vi "ReadAirmarData.vi"(8 "Error in":errorcluster, 9 "Airmar Wind Queue Cluster":T2, 10 "AirmarGPS-Compass Queue Cluster":T3, 11 "VISA UART port":refnum<visa-resource-name>) -> (0 "Error out":errorcluster, 3 "read buffer":string)   [LabVIEW 2013]
doc: "This VI reads Airmar data from the serial port, extracts the data of relevance, and writes the data to the proper queues for filtering and notification.\n\nEric Schneider, March 2014"
uses:
  Data/TypeDefs/GPS-Compass Queue Cluster.ctl
  Data/TypeDefs/UTM Location.ctl
  Data/TypeDefs/WindData Queue Cluster.ctl
  Data/TypeDefs/Notifiers.ctl
  Data/TypeDefs/Sail Set Suggestions.ctl
  Data/TypeDefs/Rudder Set Suggestions.ctl
  Data/TypeDefs/OverrideInformation.ctl
  Data/TypeDefs/OverrideMode.ctl
  Data/TypeDefs/MotorSetup.ctl
  Data/TypeDefs/DynamixelSetupInfo.ctl
  Data/TypeDefs/AirmarStatus.ctl
  Data/TypeDefs/HardwareOnline.ctl
panel:
  in  "Notifier References":T1
  out "Longitude [deg]":string
  out "Latitude [deg]":string
  in  "time zone":i32
  out "Time":string
  out "Mode":string
  out "Date [ddmmyy]":string
  out "Course over ground [degrees]":string
  out "Status":string
  out "Speed over ground [knots]":string
  out "E/W":string
  out "Longitude":string
  out "N/S":string
  out "Latitude":string
  out "UTC Time":string
  out "NMEA sentences":string
  # "[hhmmss.sss]"
  # "A = vAlid data\nV = inValid data"
  # "[ddmm.mmmm]"
  # "[dddmm.mmmm]"
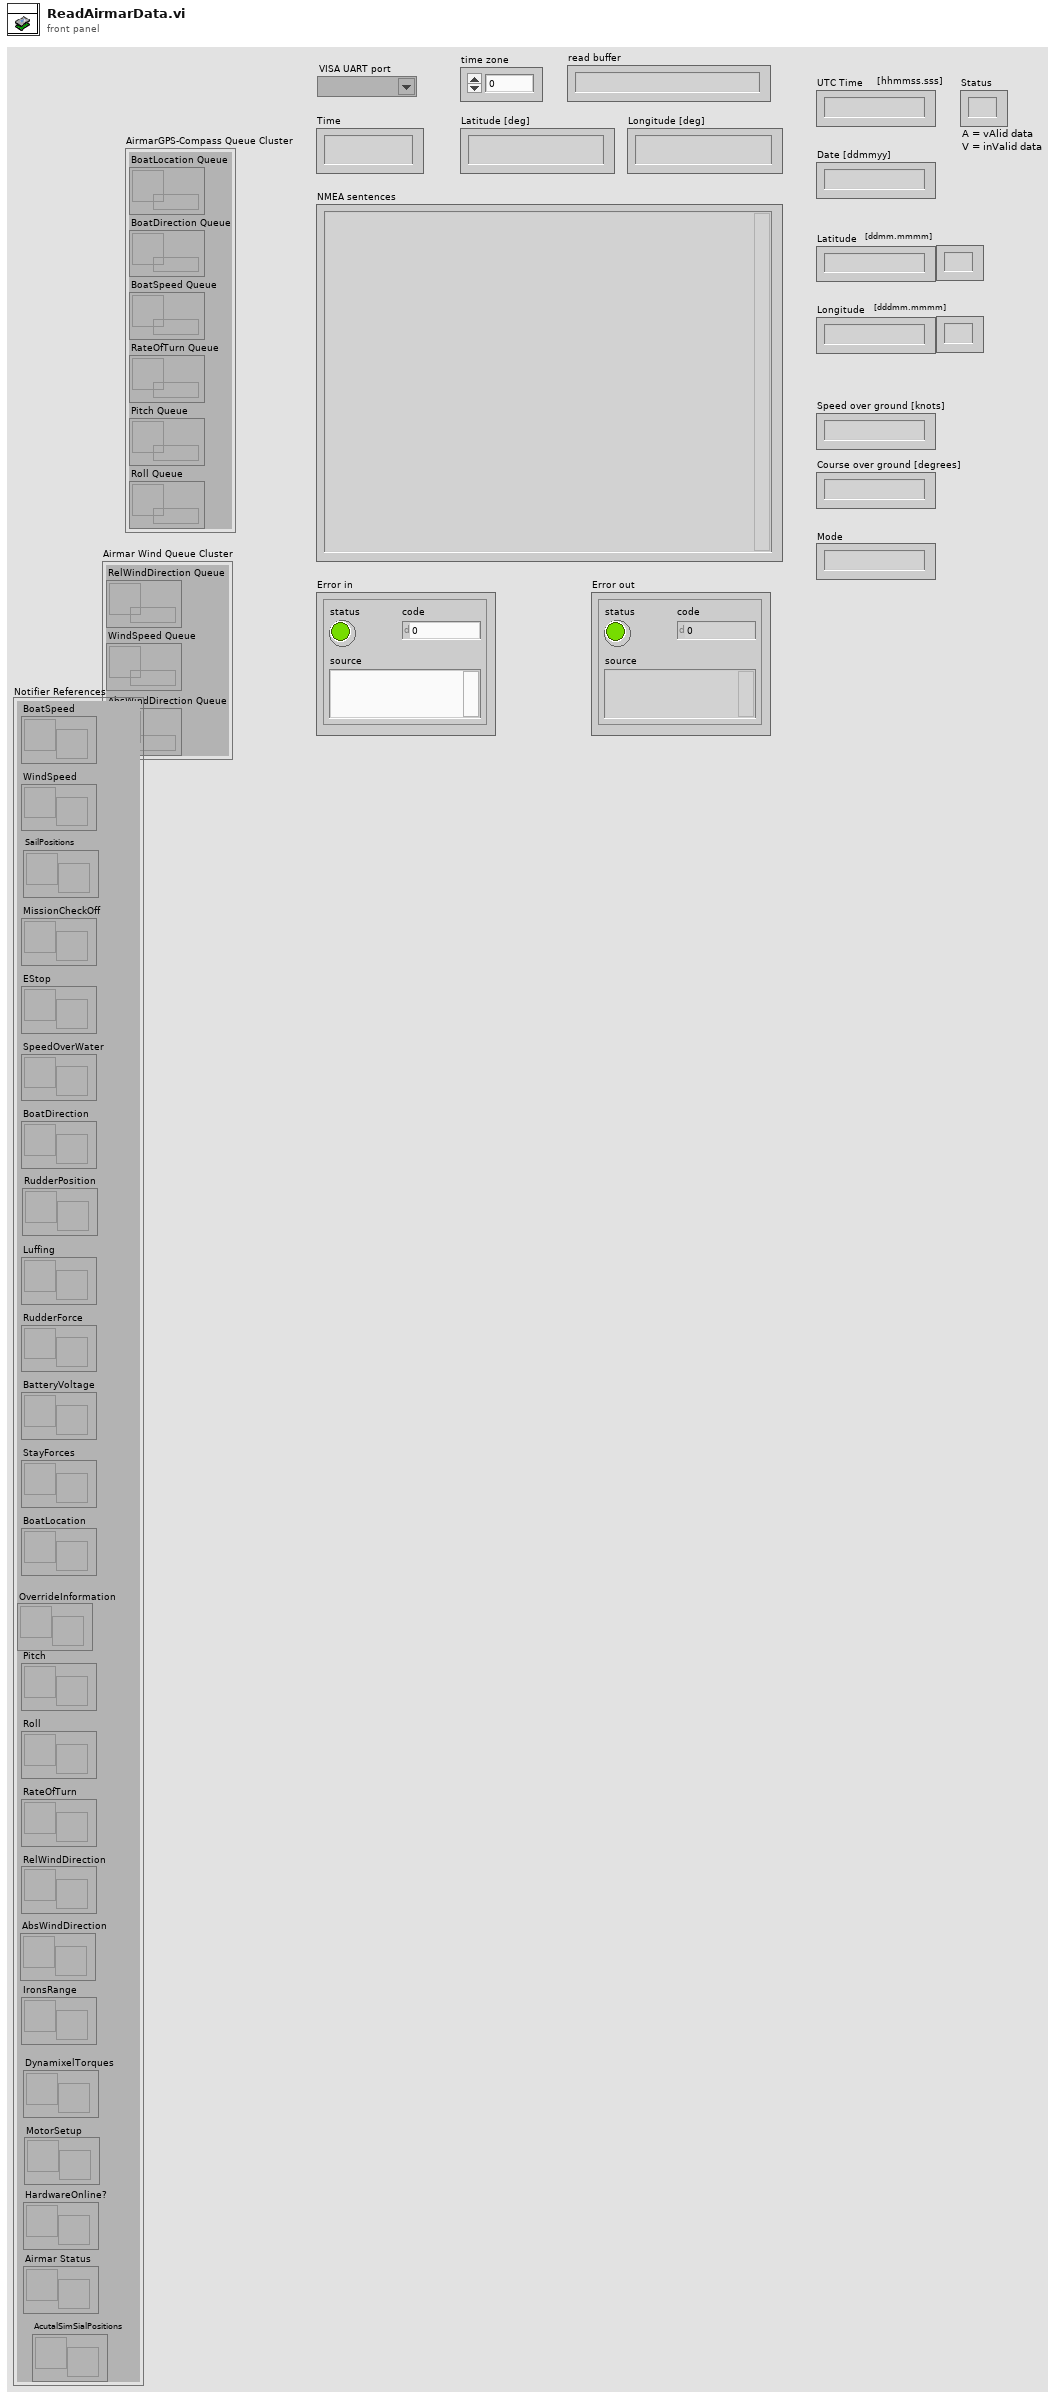
[diagram p1: front panel]
types:
  T1 = typedef "Notifiers.ctl" = cluster{"BoatSpeed":refnum<notifier>, "WindSpeed":refnum<notifier>, "MissionCheckOff":refnum<notifier>, "EStop":refnum<notifier>, "SpeedOverWater":refnum<notifier>, "BoatDirection":refnum<notifier>, "Luffing":refnum<notifier>, "RudderForce":refnum<notifier>, "BatteryVoltage":refnum<notifier>, "StayForces":refnum<notifier>, "BoatLocation":refnum<notifier>, "Pitch":refnum<notifier>, "Roll":refnum<notifier>, "RateOfTurn":refnum<notifier>, "RelWindDirection":refnum<notifier>, "SailPositions":refnum<notifier>, "RudderPosition":refnum<notifier>, "IronsRange":refnum<notifier>, "AbsWindDirection":refnum<notifier>, "OverrideInformation":refnum<notifier>, "DynamixelTorques":refnum<notifier>, "MotorSetup":refnum<notifier>, "Airmar Status":refnum<notifier>, "HardwareOnline?":refnum<notifier>, "AcutalSimSialPositions":refnum<notifier>}
  T2 = typedef "WindData Queue Cluster.ctl" = cluster{"RelWindDirection Queue":refnum<queue>, "WindSpeed Queue":refnum<queue>, "AbsWindDirection Queue":refnum<queue>}
  T3 = typedef "GPS-Compass Queue Cluster.ctl" = cluster{"BoatLocation Queue":refnum<queue>, "BoatDirection Queue":refnum<queue>, "BoatSpeed Queue":refnum<queue>, "RateOfTurn Queue":refnum<queue>, "Pitch Queue":refnum<queue>, "Roll Queue":refnum<queue>}
  T4 = typedef "AirmarStatus.ctl" = cluster{"Sensor Connected":bool, "Sensor Initialized":bool, "Sensor OK":bool, "Latest Error String":bool, "GPS Lock":bool}
  T5 = typedef "UTM Location.ctl" = cluster{"UTM Zone":dbl, "Hemisphere":enum16{"North", "South"}, "East":dbl, "North":dbl}
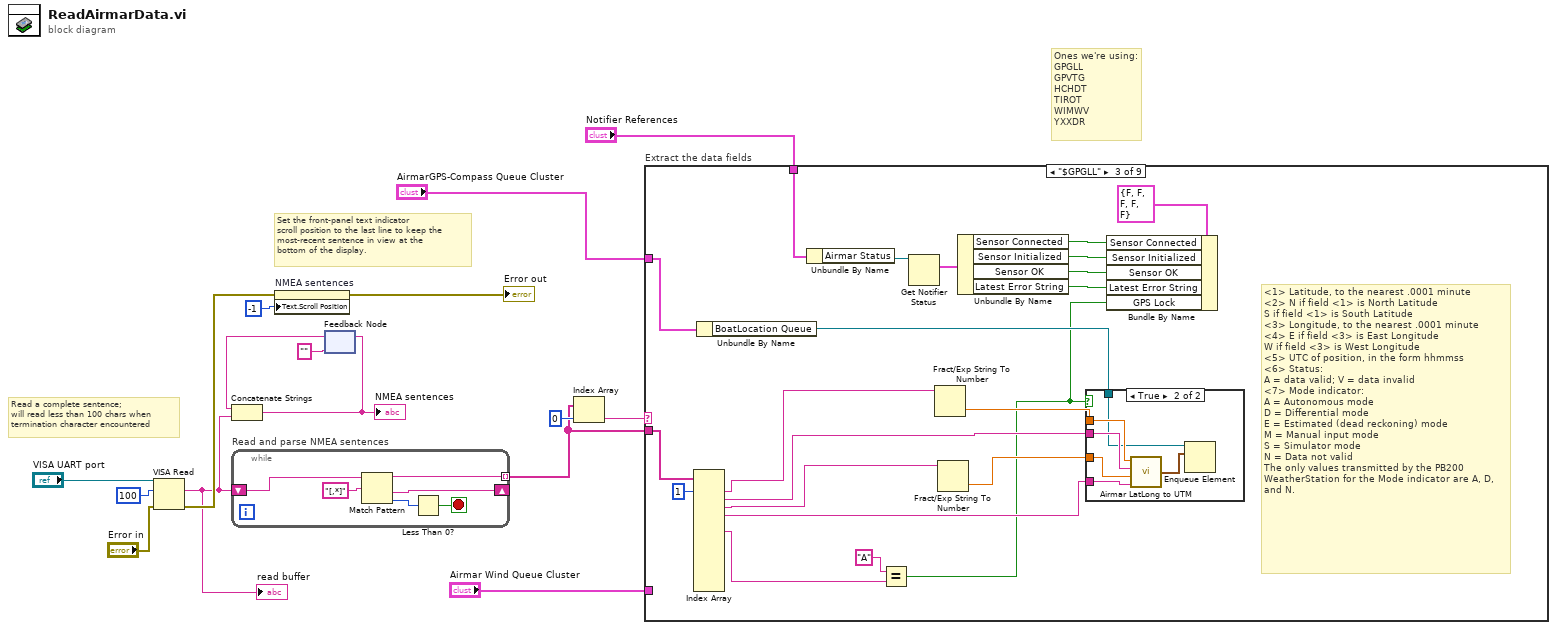
[diagram p0: block diagram]
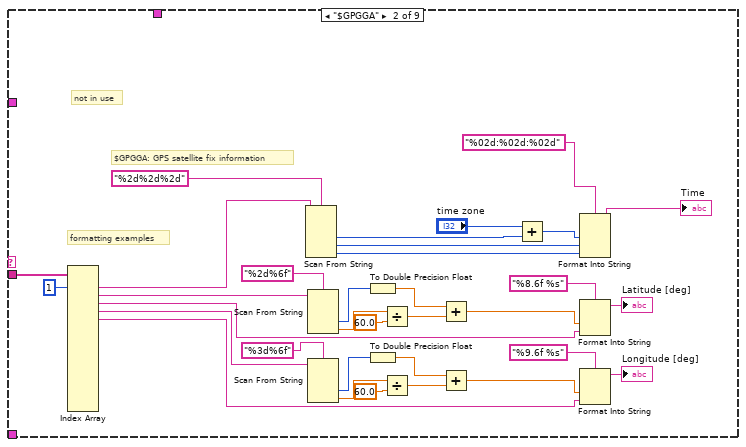
[diagram p3: hidden frame]
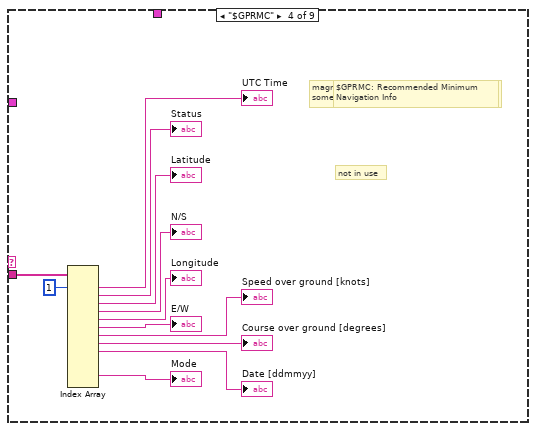
[diagram p5: hidden frame]
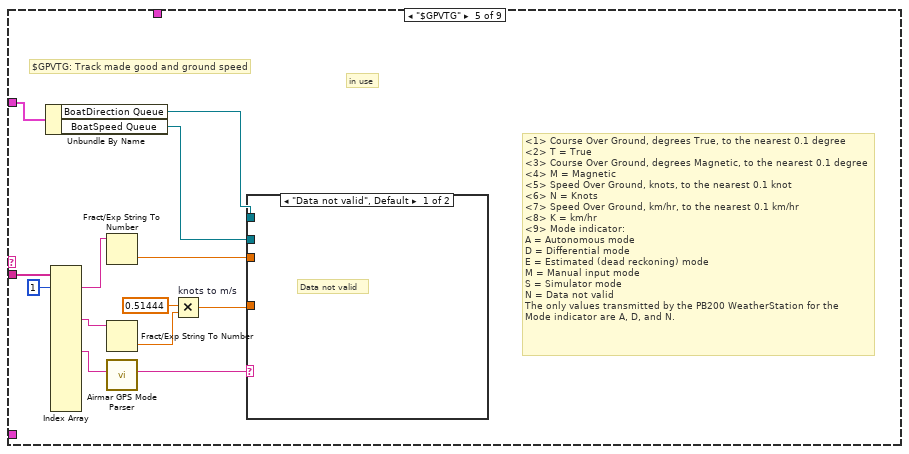
[diagram p6: hidden frame]
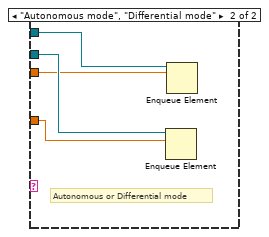
[diagram p7: hidden frame]
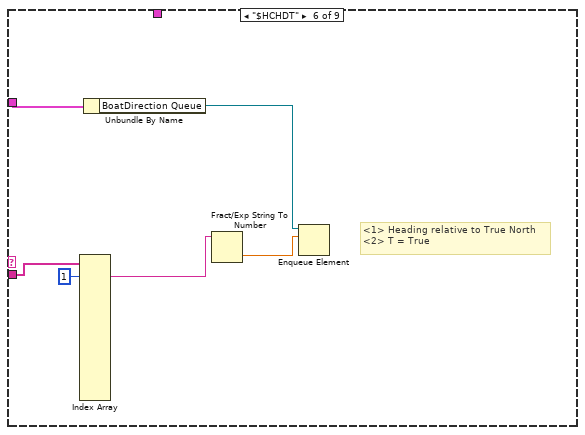
[diagram p8: hidden frame]
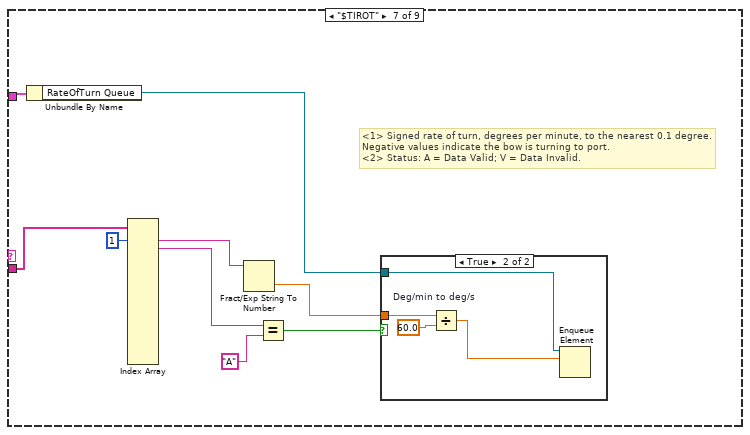
[diagram p9: hidden frame]
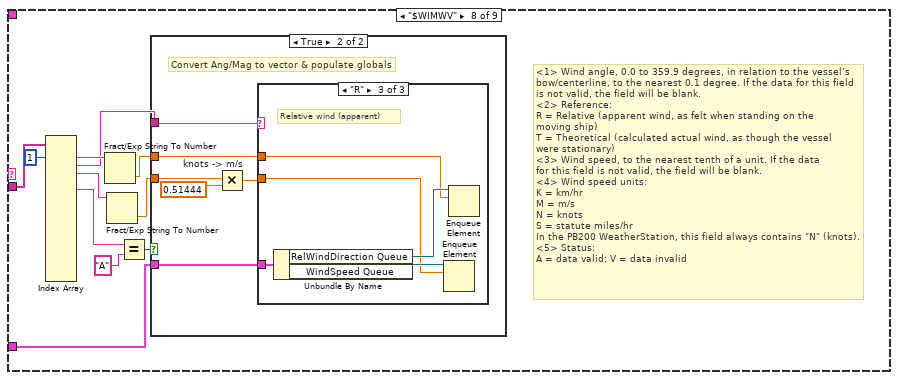
[diagram p11: hidden frame]
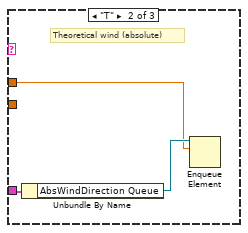
[diagram p14: hidden frame]
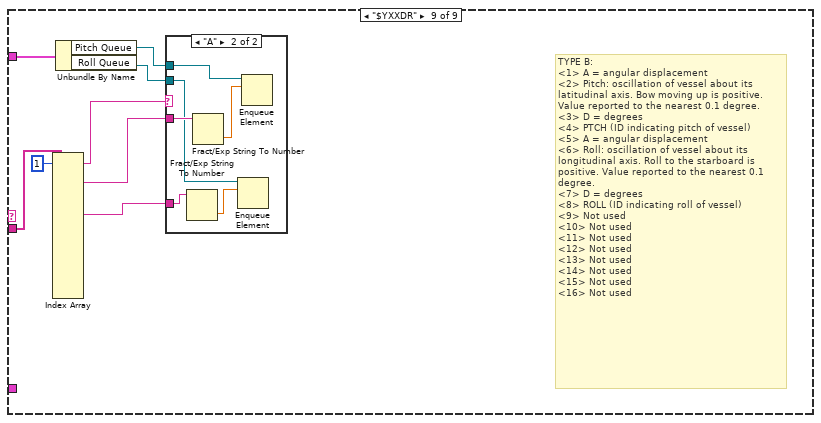
[diagram p15: hidden frame]
diagram:
  # "Ones we're using:\nGPGLL\nGPVTG\nHCHDT\nTIROT\nWIMWV\nYXXDR"
  # "Set the front-panel text indicator\nscroll position to the last line to keep the\nmost-recent sentence in view at the\nbottom of the display."
  # "Read a complete sentence;\nwill read less than 100 chars when\ntermination character encountered"
  n1 = VISA Read(VISA resource name="VISA UART port", byte count=u32 100, error in (no error)="Error in") -> (read buffer=w11:string, error out=w16:errorcluster)  [unwired: 2 out]
  "read buffer" <- w11
  n2 = while "Read and parse NMEA sentences" {
    tunnel: [w20] -> w13 mode=indexing
    shift-right: [w19] -> _
    shift-left: w11 -> [w21]
    stop <- w18 stop-if-true
    n3 = Match Pattern(string=w21, regular expression="[,*]") -> (before substring=w20:string, after substring=w19:string, offset past match=w17:i32)  [unwired: 1 in, 1 out]
    n4 = Less Than 0?(x=w17) -> (x < 0?=w18:bool)
  }
  n5 = property on="NMEA sentences" class="Str"(error in=w16, "Text.Scroll Position"=-1) -> (error out=→"Error out":errorcluster)  [unwired: 1 in, 1 out]
  n6 = feedback #1("") -> (w9:string)
  n7 = Concatenate Strings "Concatenate Strings"(w9, w11) -> (w7:string)
  "NMEA sentences" <- w7
  n8 = feedback-in #1(w7) -> ()
  n9 = Index Array "Index Array"(array=w13, index=0) -> (element=w12:string)
  n10 = case "Extract the data fields" shown="\"$GPGLL\"" w12 {
    tunnel: w13 -> [_ w55 w71 w94 w107 w117 w123 w141 w163]
    tunnel: "AirmarGPS-Compass Queue Cluster" -> [_ _ w72 _ w97 w114 w126 _ w161]
    tunnel: "Airmar Wind Queue Cluster" -> [_ _ _ _ _ _ _ w135 _]
    tunnel: "Notifier References" -> [_ _ w63 _ _ _ _ _ _]
    frame Default {
      # "Unknown sentence."
    }
    frame "$GPGGA" {
      # "not in use"
      # "formatting examples"
      # "$GPGGA: GPS satellite fix information"
      n11 = Index Array "Index Array"(array=w55, index #1=1 ("index")) -> (element #1=w52:string, element #2=w43:string, element #3=w35:string, element #4=w24:string, element #5=w23:string)  [unwired: 15 in, 11 out]
      n12 = Scan From String "Scan From String"(format string="%2d%2d%2d", input string=w52) -> (output 1=w45:i32, output 2=w48:i32, output 3=w50:i32)  [unwired: 5 in, 3 out]
      n13 = Scan From String(format string="%2d%6f", input string=w43) -> (output 1=w40:i32, output 2=w42:dbl)  [unwired: 4 in, 3 out]
      n14 = Scan From String(format string="%3d%6f", input string=w24) -> (output 1=w28:i32, output 2=w26:dbl)  [unwired: 4 in, 3 out]
      n15 = To Double Precision Float(number=w40) -> (double precision float=w38:dbl)
      n16 = To Double Precision Float(number=w28) -> (double precision float=w30:dbl)
      n17 = Divide(x=w42, y=60.0) -> (x/y=w39:dbl)
      n18 = Divide(x=w26, y=60.0) -> (x/y=w29:dbl)
      n19 = Add(x=w38, y=w39) -> (x+y=w36:dbl)
      n20 = Add(x=w30, y=w29) -> (x+y=w32:dbl)
      n21 = Add(x="time zone", y=w45) -> (x+y=w46:i32)
      n22 = Format Into String "Format Into String"(format string="%02d:%02d:%02d", w46, w48, w50) -> (resulting string=→"Time":string)  [unwired: 2 in, 1 out]
      n23 = Format Into String(format string="%8.6f %s", w36, w35) -> (resulting string=→"Latitude [deg]":string)  [unwired: 2 in, 1 out]
      n24 = Format Into String(format string="%9.6f %s", w32, w23) -> (resulting string=→"Longitude [deg]":string)  [unwired: 2 in, 1 out]
    }
    frame "$GPGLL" {
      # "<1> Latitude, to the nearest .0001 minute\n<2> N if field <1> is North Latitude\nS if field <1> is South Latitude\n<3> Longitude, to the nearest .0001 minute\n<4> E if field <3> is East Longitude\nW if field <3> is West Longitude\n<5> UTC of position, in the form hhmmss\n<6> Status:\nA = data valid; V = data invalid\n<7> Mode indicator:\nA = Autonomous mode\nD = Differential mode\nE = Estimated (dead reckoning) mode\nM = Manual input mode\nS = Simulator mode\nN = Data not valid\nThe only values transmitted by the PB200 WeatherStation for the Mode indicator are A, D, and N."
      n25 = Index Array "Index Array"(array=w71, index #1=1 ("index")) -> (element #1=w70:string, element #2=w69:string, element #3=w68:string, element #4=w67:string, element #6=w66:string)  [unwired: 12 in, 8 out]
      n26 = Unbundle By Name(w72) -> ("BoatLocation Queue"=w75:refnum<queue>)
      n27 = Unbundle By Name(w63) -> ("Airmar Status"=w62:refnum<notifier>)
      n28 = Equal?(x="A" ("y"), y=w66) -> (x = y?=w60:bool)
      n29 = Get Notifier Status(notifier=w62) -> (current notification=w61:T4)  [unwired: 1 in, 4 out]
      n30 = Fract/Exp String To Number(string=w70) -> (number=w73:dbl)  [unwired: 3 in, 1 out]
      n31 = Fract/Exp String To Number(string=w68) -> (number=w74:dbl)  [unwired: 3 in, 1 out]
      n32 = Unbundle By Name(w61) -> ("Sensor Connected"=w56:bool, "Sensor Initialized"=w57:bool, "Sensor OK"=w58:bool, "Latest Error String"=w59:bool)
      n33 = case shown="True" w60 {
        tunnel: w69 -> [_ w82]
        tunnel: w74 -> [_ w81]
        tunnel: w67 -> [_ w80]
        tunnel: w75 -> [_ w78]
        tunnel: w73 -> [_ w79]
        frame False {
        }
        frame True {
          n34 = call "Airmar LatLong to UTM.vi"("East/West"=w80, "Longitude"=w81, "North/South"=w82, "Latitude"=w79) -> ("Robot UTM Location"=w77:T5)
          n35 = Enqueue Element(queue=w78, element=w77) -> ()  [unwired: 2 in, 3 out]
        }
      }
      n36 = Bundle By Name(cluster=T4 {"Sensor Connected"=FALSE, "Sensor Initialized"=FALSE, "Sensor OK"=FALSE, "Latest Error String"=FALSE, "GPS Lock"=FALSE}, "Sensor Connected"=w56, "Sensor Initialized"=w57, "Sensor OK"=w58, "Latest Error String"=w59, "GPS Lock"=w60) -> ()  [unwired: 1 out]
    }
    frame "$GPRMC" {
      # "not in use"
      # "magnetic variation not available w/o\nsome firmware upgrade from GlobalTop"
      # "$GPRMC: Recommended Minimum\nNavigation Info"
      n37 = Index Array "Index Array"(array=w94, index #1=1 ("index")) -> (element #1=→"UTC Time":string, element #2=→"Status":string, element #3=→"Latitude":string, element #4=→"N/S":string, element #5=→"Longitude":string, element #6=→"E/W":string, element #7=→"Speed over ground [knots]":string, element #8=→"Course over ground [degrees]":string, element #9=→"Date [ddmmyy]":string, element #12=→"Mode":string)  [unwired: 12 in, 3 out]
    }
    frame "$GPVTG" {
      # "<1> Course Over Ground, degrees True, to the nearest 0.1 degree\n<2> T = True\n<3> Course Over Ground, degrees Magnetic, to the nearest 0.1 degree\n<4> M = Magnetic\n<5> Speed Over Ground, knots, to the nearest 0.1 knot\n<6> N = Knots\n<7> Speed Over Ground, km/hr, to the nearest 0.1 km/hr\n<8> K = km/hr\n<9> Mode indicator:\nA = Autonomous mode\nD = Differential mode\nE = Estimated (dead reckoning) mode\nM = Manual input mode\nS = Simulator mode\nN = Data not valid\nThe only values transmitted by the PB200 WeatherStation for the\nMode indicator are A, D, and N."
      # "in use"
      # "$GPVTG: Track made good and ground speed"
      n38 = Unbundle By Name(w97) -> ("BoatDirection Queue"=w96:refnum<queue>, "BoatSpeed Queue"=w95:refnum<queue>)
      n39 = Index Array(array=w107, index #1=1 ("index")) -> (element #1=w105:string, element #5=w104:string, element #9=w103:string)  [unwired: 15 in, 13 out]
      n40 = Fract/Exp String To Number(string=w105) -> (number=w102:dbl)  [unwired: 3 in, 1 out]
      n41 = Fract/Exp String To Number(string=w104) -> (number=w100:dbl)  [unwired: 3 in, 1 out]
      n42 = call "Airmar GPS Mode Parser.vi"("GPS Mode (Char)"=w103) -> ("GPS Mode (Description)"=w98:string)  [unwired: 6 in]
      n43 = Multiply "knots to m/s"(x=0.51444 ("y"), y=w100) -> (x*y=w101:dbl)
      n44 = case shown="\"Data not valid\", Default" w98 {
        tunnel: w102 -> [_ w109]
        tunnel: w101 -> [_ w108]
        tunnel: w96 -> [_ w111]
        tunnel: w95 -> [_ w110]
        frame "Data not valid", Default {
          # "Data not valid"
        }
        frame "Autonomous mode", "Differential mode" {
          # "Autonomous or Differential mode"
          n45 = Enqueue Element(queue=w110, element=w108) -> ()  [unwired: 2 in, 3 out]
          n46 = Enqueue Element(queue=w111, element=w109) -> ()  [unwired: 2 in, 3 out]
        }
      }
    }
    frame "$HCHDT" {
      # "<1> Heading relative to True North\n<2> T = True"
      n47 = Index Array(array=w117, index #1=1 ("index")) -> (element #1=w116:string)  [unwired: 15 in, 15 out]
      n48 = Unbundle By Name(w114) -> ("BoatDirection Queue"=w113:refnum<queue>)
      n49 = Fract/Exp String To Number(string=w116) -> (number=w115:dbl)  [unwired: 3 in, 1 out]
      n50 = Enqueue Element(queue=w113, element=w115) -> ()  [unwired: 2 in, 3 out]
    }
    frame "$TIROT" {
      # "<1> Signed rate of turn, degrees per minute, to the nearest 0.1 degree.\nNegative values indicate the bow is turning to port.\n<2> Status: A = Data Valid; V = Data Invalid."
      n51 = Unbundle By Name(w126) -> ("RateOfTurn Queue"=w119:refnum<queue>)
      n52 = Index Array(array=w123, index #1=1 ("index")) -> (element #1=w122:string, element #2=w120:string)  [unwired: 15 in, 14 out]
      n53 = Fract/Exp String To Number(string=w122) -> (number=w124:dbl)  [unwired: 3 in, 1 out]
      n54 = Equal?(x=w120, y="A") -> (x = y?=w125:bool)
      n55 = case shown="True" w125 {
        tunnel: w124 -> [_ w130]
        tunnel: w119 -> [_ w127]
        frame False {
        }
        frame True {
          n56 = Divide "Deg/min to deg/s"(x=w130, y=60.0) -> (x/y=w128:dbl)
          n57 = Enqueue Element(queue=w127, element=w128) -> ()  [unwired: 2 in, 3 out]
        }
      }
    }
    frame "$WIMWV" {
      # "<1> Wind angle, 0.0 to 359.9 degrees, in relation to the vessel’s\nbow/centerline, to the nearest 0.1 degree. If the data for this field\nis not valid, the field will be blank.\n<2> Reference:\nR = Relative (apparent wind, as felt when standing on the\nmoving ship)\nT = Theoretical (calculated actual wind, as though the vessel\nwere stationary)\n<3> Wind speed, to the nearest tenth of a unit. If the data\nfor this field is not valid, the field will be blank.\n<4> Wind speed units:\nK = km/hr\nM = m/s\nN = knots\nS = statute miles/hr\nIn the PB200 WeatherStation, this field always contains \"N\" (knots).\n<5> Status:\nA = data valid; V = data invalid"
      n58 = Index Array(array=w141, index #1=1 ("index")) -> (element #1=w139:string, element #2=w136:string, element #3=w138:string, element #5=w137:string)  [unwired: 15 in, 12 out]
      n59 = Fract/Exp String To Number(string=w139) -> (number=w134:dbl)  [unwired: 3 in, 1 out]
      n60 = Fract/Exp String To Number(string=w138) -> (number=w133:dbl)  [unwired: 3 in, 1 out]
      n61 = Equal?(x=w137, y="A") -> (x = y?=w132:bool)
      n62 = case shown="True" w132 {
        tunnel: w133 -> [_ w144]
        tunnel: w134 -> [_ w147]
        tunnel: w136 -> [_ w146]
        tunnel: w135 -> [_ w142]
        frame False {
        }
        frame True {
          # "Convert Ang/Mag to vector & populate globals"
          n63 = Multiply "knots -> m/s"(x=w144, y=0.51444) -> (x*y=w145:dbl)
          n64 = case shown="\"R\"" w146 {
            tunnel: w145 -> [_ _ w151]
            tunnel: w147 -> [_ w148 w153]
            tunnel: w142 -> [_ w150 w155]
            frame "", Default {
            }
            frame "T" {
              # "Theoretical wind (absolute)"
              n65 = Unbundle By Name(w150) -> ("AbsWindDirection Queue"=w149:refnum<queue>)
              n66 = Enqueue Element(queue=w149, element=w148) -> ()  [unwired: 2 in, 3 out]
            }
            frame "R" {
              # "Relative wind (apparent)"
              n67 = Unbundle By Name(w155) -> ("RelWindDirection Queue"=w154:refnum<queue>, "WindSpeed Queue"=w152:refnum<queue>)
              n68 = Enqueue Element(queue=w152, element=w151) -> ()  [unwired: 2 in, 3 out]
              n69 = Enqueue Element(queue=w154, element=w153) -> ()  [unwired: 2 in, 3 out]
            }
          }
        }
      }
    }
    frame "$YXXDR" {
      # "TYPE B:\n<1> A = angular displacement\n<2> Pitch: oscillation of vessel about its latitudinal axis. Bow moving up is positive. Value reported to the nearest 0.1 degree.\n<3> D = degrees\n<4> PTCH (ID indicating pitch of vessel)\n<5> A = angular displacement\n<6> Roll: oscillation of vessel about its longitudinal axis. Roll to the starboard is positive. Value reported to the nearest 0.1 degree.\n<7> D = degrees\n<8> ROLL (ID indicating roll of vessel)\n<9> Not used\n<10> Not used\n<11> Not used\n<12> Not used\n<13> Not used\n<14> Not used\n<15> Not used\n<16> Not used"
      n70 = Index Array(array=w163, index #1=1 ("index")) -> (element #1=w162:string, element #2=w157:string, element #6=w156:string)  [unwired: 15 in, 13 out]
      n71 = Unbundle By Name(w161) -> ("Pitch Queue"=w160:refnum<queue>, "Roll Queue"=w159:refnum<queue>)
      n72 = case shown="\"A\"" w162 {
        tunnel: w157 -> [_ w169]
        tunnel: w156 -> [_ w168]
        tunnel: w160 -> [_ w166]
        tunnel: w159 -> [_ w164]
        frame "", Default {
        }
        frame "A" {
          n73 = Fract/Exp String To Number(string=w168) -> (number=w165:dbl)  [unwired: 3 in, 1 out]
          n74 = Fract/Exp String To Number(string=w169) -> (number=w167:dbl)  [unwired: 3 in, 1 out]
          n75 = Enqueue Element(queue=w164, element=w165) -> ()  [unwired: 2 in, 3 out]
          n76 = Enqueue Element(queue=w166, element=w167) -> ()  [unwired: 2 in, 3 out]
        }
      }
    }
  }
